vi "DynamicObject.vi"(9 "h":dbl, 10 "P0":dbl, 11 "Cluster in":cluster{"P1":dbl, "P2":dbl, "P3":dbl}) -> (3 "Cluster out":cluster{"P1":dbl, "P2":dbl, "P3":dbl})   [LabVIEW 2017]
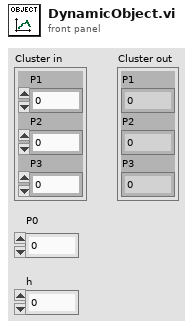
[diagram p1: front panel]
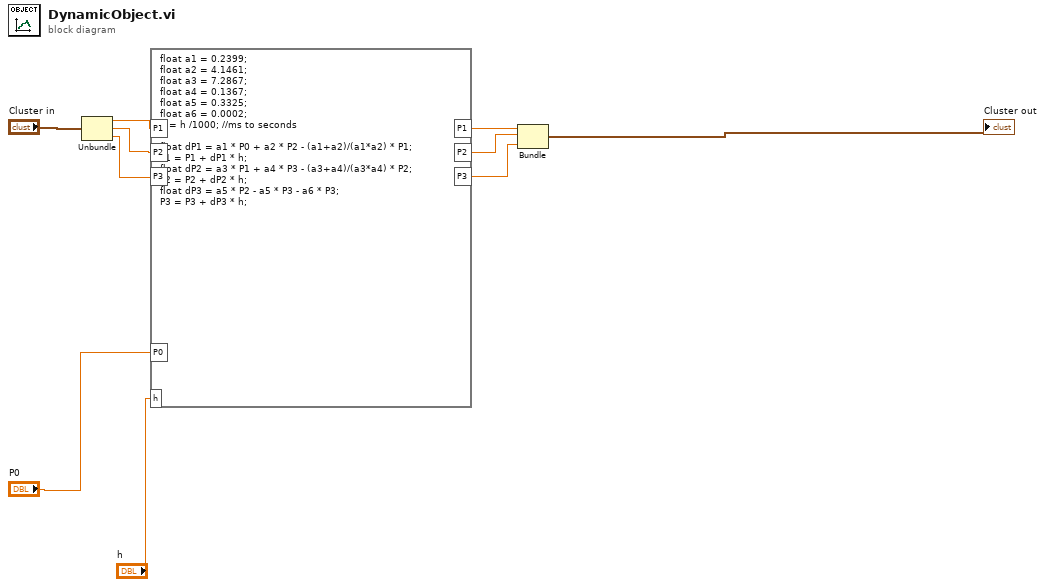
[diagram p0: block diagram]
diagram:
  n1 = Unbundle("Cluster in") -> ("P1"=w7:dbl, "P2"=w8:dbl, "P3"=w9:dbl)
  n2 = formula code="float a1 = 0.2399;\nfloat a2 = 4.1461;\nfloat a3 = 7.2867;\nfloat a4 = 0.1367;\nfloat a5 = 0.3325;\nfloat a6 = 0.0002;\nh = h /1000; //ms to seconds\n\nfloat dP1 = a1 * P0 + a2 * P2 - (a1+a2)/(a1*a2) * P1;\nP1 = P1 + dP1 * h;\nfloat dP2 = a3 * P1 + a4 * P3 - (a3+a4)/(a3*a4) * P2;\nP2 = P2 + dP2 * h;\nfloat dP3 = a5 * P2 - a5 * P3 - a6 * P3;\nP3 = P3 + dP3 * h;"("P0"="P0", "P1"=w7, "P2"=w8, "P3"=w9, "h"="h") -> ("P1"=w3:dbl, "P2"=w4:dbl, "P3"=w5:dbl)
  n3 = Bundle("P1"=w3, "P2"=w4, "P3"=w5) -> (→"Cluster out":cluster{"P1":dbl, "P2":dbl, "P3":dbl})  [unwired: 1 in]
